vi "WIP_Script.vi"(11 "WIP Limit":T1) -> (3 "iNSERT Script":string)   [LabVIEW 2020]
uses:
  Controls/WIP Limit.ctl
  Controls/WIP_old.ctl
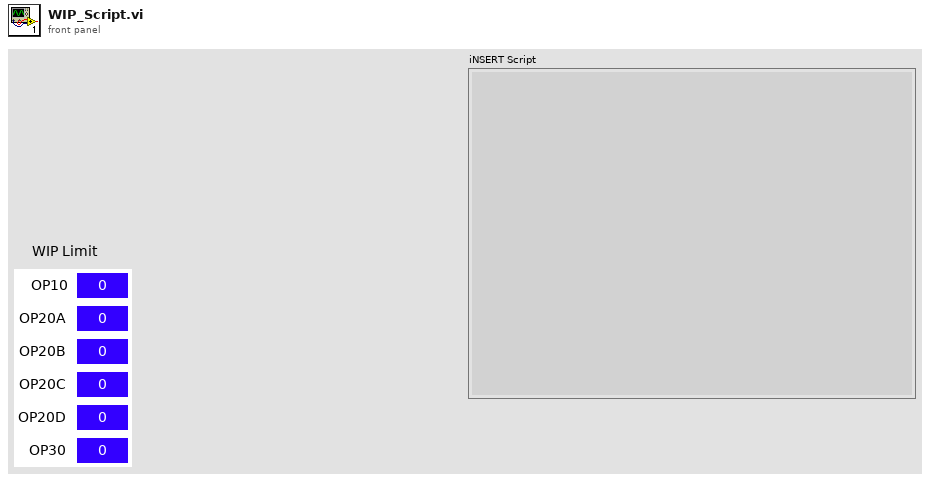
[diagram p1: front panel]
types:
  T1 = typedef "WIP Limit.ctl" = cluster{"OP10":T2, "OP20A":T2, "OP20B":T2, "OP20C":T2, "OP20D":T2, "OP30":T2}
  T2 = typedef "WIP_old.ctl" = i64
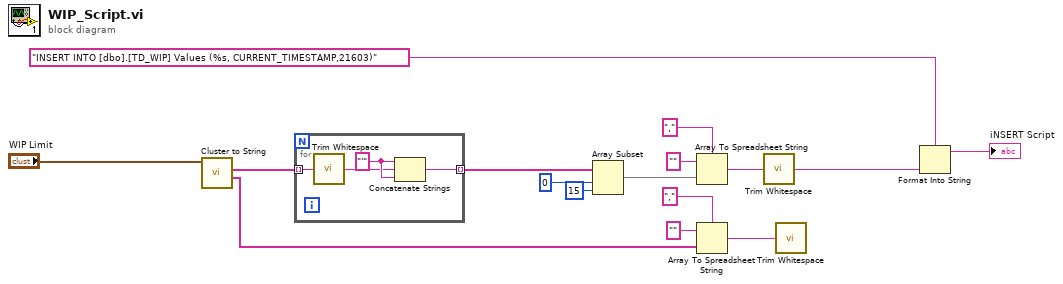
[diagram p0: block diagram]
diagram:
  n1 = call <userlib>:"Cluster to String.vi"("Variant In"="WIP Limit") -> ("Format String Name"=w10:string[], "Format String Array"=w2:string[])  [unwired: 7 in, 2 out]
  n2 = for {
    tunnel: w2 -> [w20] mode=indexing
    tunnel: [w18] -> w1 mode=indexing
    w19 = "'" ("string")
    n3 = call <vilib>:"Trim Whitespace.vi"("string"=w20) -> ("trimmed string"=w17:string)  [unwired: 1 in]
    n4 = Concatenate Strings(w19, w17, w19) -> (w18:string)
  }
  n5 = Array Subset(array=w1, index=0, length=15) -> (w8:string[])
  n6 = Array To Spreadsheet String(delimiter (Tab)=",", array=w8, 3:"" ("format string")) -> (spreadsheet string=w5:string)
  n7 = Array To Spreadsheet String(delimiter (Tab)=",", array=w10, 3:"" ("format string")) -> (spreadsheet string=w13:string)
  n8 = call <vilib>:"Trim Whitespace.vi"("string"=w5) -> ("trimmed string"=w3:string)  [unwired: 1 in]
  n9 = call <vilib>:"Trim Whitespace.vi"("string"=w13) -> ()  [unwired: 1 in, 1 out]
  n10 = Format Into String(format string="INSERT INTO [dbo].[TD_WIP] Values (%s, CURRENT_TIMESTAMP,21603)", w3) -> (resulting string=→"iNSERT Script":string)  [unwired: 2 in, 1 out]
